vi "Set Fetch Step Values.vi"(8 "error in (no error)":errorcluster, 11 "Skyworks - 2G PVT in":refnum<class "Skyworks - PVT.lvclass">) -> (0 "error out":errorcluster, 2 "Fetch Step Out":refnum<k7>, 3 "Skyworks - 2G PVT out":refnum<class "Skyworks - PVT.lvclass">)   [LabVIEW 2018, in "Skyworks PVT.lvlib" / "Skyworks - PVT.lvclass"]
uses:
  Skyworks - PVT.lvclass
  C:/Sequence Automation/Plugins/Measurement Interface.lvlibp/Measurement Interface.lvclass
  Skyworks - PVT.lvclass/Skyworks - PVT.ctl
  Plugins/Measurement Interface.lvlibp/Private Methods/Engine Reference/Read Engine Reference.vi
  Plugins/Measurement Interface.lvlibp/Private Methods/Measurement Name/Read Measurement Name.vi
  Plugins/TestStand API Tools (TSAT).lvlibp/Step Actions/TSAT Step Actions.lvlib
  Plugins/Measurement Interface.lvlibp/Measurement Interface.lvclass
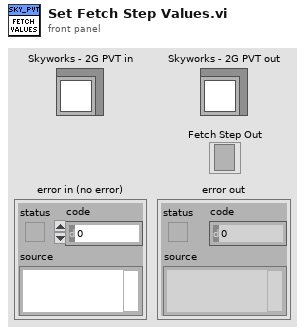
[diagram p1: front panel]
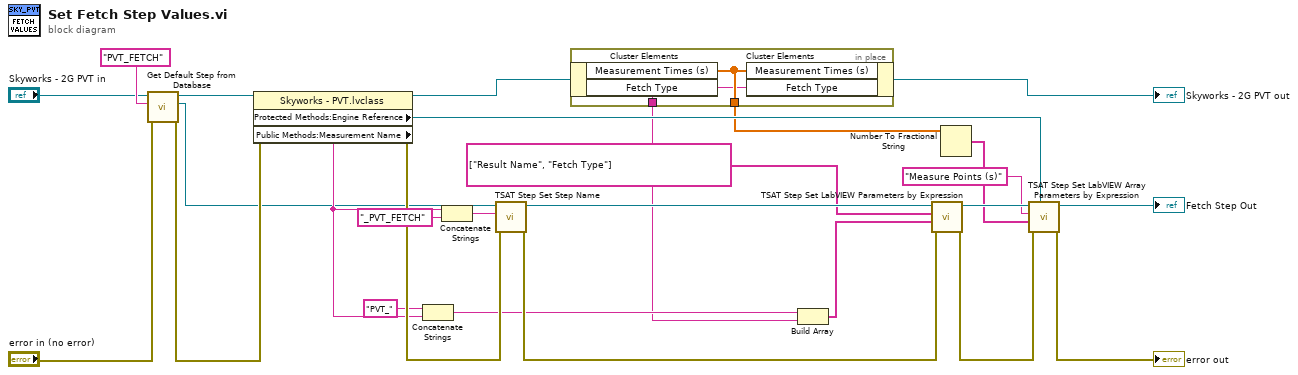
[diagram p0: block diagram]
diagram:
  n1 = call "Get Default Step from Database.vi"("error in (no error)"="error in (no error)", "Default Step"="PVT_FETCH", "Measurement Interface in"="Skyworks - 2G PVT in") -> ("error out"=w2:errorcluster, "Cloned Step"=w1:refnum<k7>, "Measurement Interface out"=w4:refnum<class "Skyworks - PVT.lvclass">)  [unwired: 6 in]
  n2 = property class="Skyworks - PVT.lvclass"(reference=w4, error in=w2) -> (reference out=w10:refnum<class "Skyworks - PVT.lvclass">, error out=w27:errorcluster, "Protected Methods:Engine Reference"=w24:refnum<k7>, "Public Methods:Measurement Name"=w13:string)
  n3 = Concatenate Strings("PVT_" ("string"), w13) -> (w15:string)
  n4 = Concatenate Strings(w13, "_PVT_FETCH" ("string")) -> (w26:string)
  n5 = call "TSAT Step Set Step Name.vi"("Error In"=w27, "Name"=w26, "Step In"=w1) -> ("Error Out"=w21:errorcluster, "Step Out"=w20:refnum<k7>)  [unwired: 7 in]
  n6 = in-place {
    in-place-border: [w29] -> w8
    in-place-border: [w28] -> w7
    n7 = in-place-cluster #1(w10) -> ("Measurement Times (s)"=w29:dbl[], "Fetch Type"=w28:string)
    n8 = in-place-cluster #1("Measurement Times (s)"=w29, "Fetch Type"=w28) -> (→"Skyworks - 2G PVT out":refnum<class "Skyworks - PVT.lvclass">)
  }
  n9 = Build Array(w15, w7) -> (w14:string[])
  n10 = call "TSAT Step Set LabVIEW Parameters by Expression.vi"("Error In"=w21, "Value Expressions"=w14, "Parameters to Set"=string[] ["Result Name", "Fetch Type"], "Step In"=w20) -> ("Error Out"=w18:errorcluster, "Step Out"=w19:refnum<k7>)  [unwired: 6 in]
  n11 = Number To Fractional String(number=w8) -> (F-format string=w11:string[])  [unwired: 3 in]
  n12 = call "TSAT Step Set LabVIEW Array Parameters by Expression.vi"("Engine In"=w24, "Error In"=w18, "Value Expressions"=w11, "Parameter to Set"="Measure Points (s)", "Step In"=w19) -> ("Error Out"=→"error out":errorcluster, "Step Out"=→"Fetch Step Out":refnum<k7>)  [unwired: 5 in]
